vi "dinamometro.vi"() -> ()   [LabVIEW 2009]
panel:
  out "output string":string
  in  "VISA resource name":refnum<visa-resource-name>
  out "x-y":u32
  out "Numeric":i32
  in  "stop":bool
  out "read buffer":string
  out "error out":errorcluster
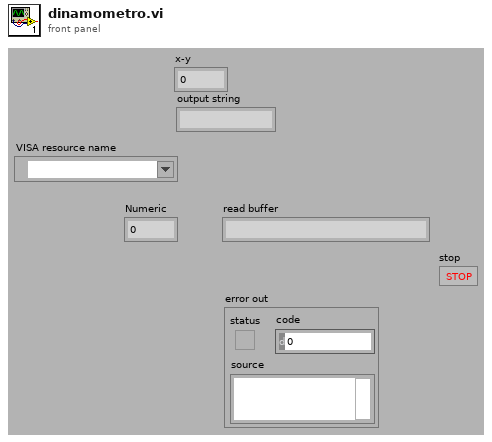
[diagram p1: front panel]
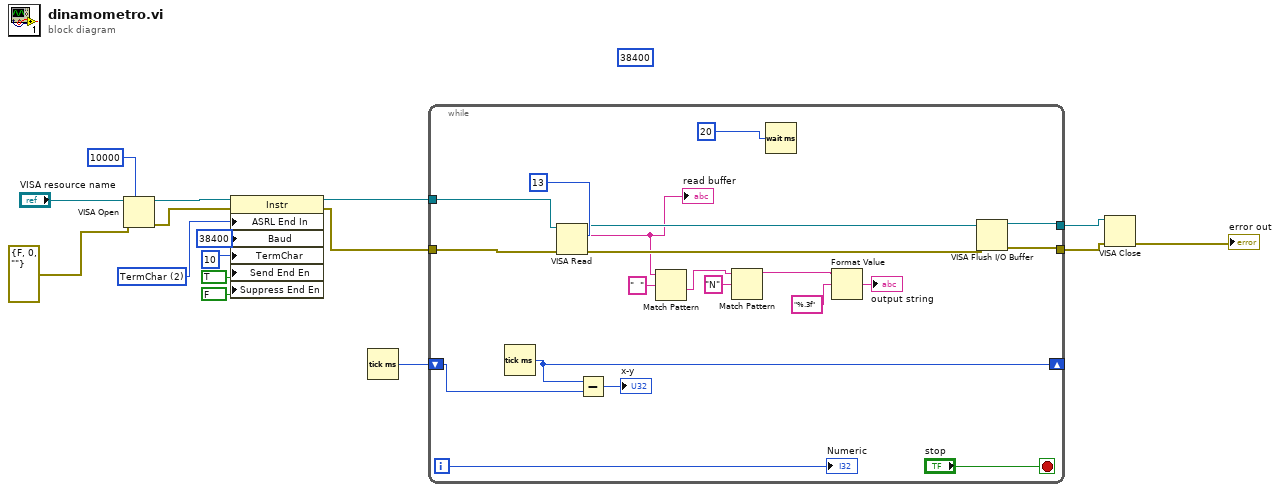
[diagram p0: block diagram]
diagram:
  w10 = u16 2 items=["None", "Last Bit", "TermChar"] ("Serial Settings:End Mode for Reads")
  (unwired) u32 38400 ("baud rate (9600)")
  n1 = VISA Open(timeout (0)=u32 10000 ("VISA Open timeout (0)"), error in (no error)=errorcluster {"status"=FALSE, "code"=0, "source"=""}, VISA resource name="VISA resource name") -> (VISA resource name=w12:refnum<visa-resource-name>, error out=w11:errorcluster)  [unwired: 2 in]
  n2 = property class="Instr"(reference=w12, error in=w11, "ASRL End In"=w10, "Baud"=u32 38400 ("Serial Settings:Baud Rate"), "TermChar"=u8 10 ("Message Based Settings:Termination Character"), "Send End En"=TRUE ("Message Based Settings:Send End Enable"), "Suppress End En"=FALSE ("Message Based Settings:Suppress End Enable")) -> (reference out=w2:refnum<visa-resource-name>, error out=w1:errorcluster)
  n3 = Tick Count (ms)() -> (millisecond timer value=w16:u32)
  n4 = while {
    shift-right: [w32] -> _
    shift-left: w16 -> [w33]
    tunnel: [w26] -> w4
    tunnel: [w27] -> w3
    tunnel: w2 -> [w30]
    tunnel: w1 -> [w29]
    i -> [w34]
    stop <- "stop" stop-if-true
    n5 = Tick Count (ms)() -> (millisecond timer value=w32:u32)
    n6 = VISA Read(VISA resource name=w30, byte count=u32 13, error in (no error)=w29) -> (VISA resource name out=w25:refnum<visa-resource-name>, read buffer=w18:string, error out=w24:errorcluster)  [unwired: 1 out]
    "read buffer" <- w18
    n7 = Subtract(x=w32, y=w33) -> (x-y=→"x-y":u32)
    n8 = Match Pattern(string=w18, regular expression="  ") -> (after substring=w17:string)  [unwired: 1 in, 3 out]
    n9 = Match Pattern(string=w17, regular expression="N") -> (before substring=w22:string)  [unwired: 1 in, 3 out]
    n10 = Wait (ms)(milliseconds to wait=u32 20) -> ()  [unwired: 1 out]
    n11 = Format Value(string ("")=w22, format string="%.3f") -> (output string=→"output string":string)  [unwired: 1 in]
    n12 = VISA Flush I/O Buffer(VISA resource name=w25, error in (no error)=w24) -> (VISA resource name out=w27:refnum<visa-resource-name>, error out=w26:errorcluster)  [unwired: 1 in]
    "Numeric" <- w34
  }
  n13 = VISA Close(VISA resource name=w3, error in (no error)=w4) -> (error out=→"error out":errorcluster)
